vi "Create Table.vi"(8 "error in (no error)":errorcluster, 11 "User DB in":refnum<class "User DB.lvclass">) -> (0 "error out":errorcluster, 3 "User DB out":refnum<class "User DB.lvclass">)   [LabVIEW 2020, in "Summer of LabVIEW.lvlib" / "User DB.lvclass"]
uses:
  User DB.lvclass
  User DB.lvclass/User DB.ctl
  <vilib>/drjdpowell/SQLite Library/SQL Connection/Execute SQL (No results).vi
  SQLite/SQLite.lvclass
  <vilib>/drjdpowell/SQLite Library/SQLite.lvlib
  <vilib>/drjdpowell/SQLite Library/SQL Connection/Connection.lvclass
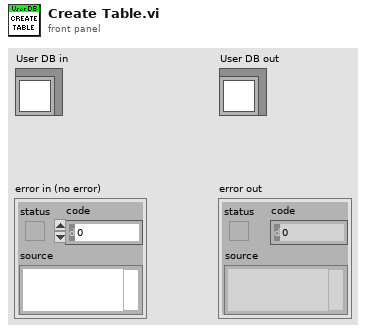
[diagram p1: front panel]
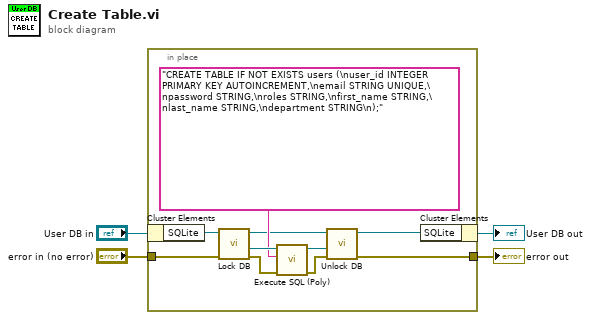
[diagram p0: block diagram]
diagram:
  n1 = in-place {
    in-place-border: "error in (no error)" -> [w13]
    in-place-border: [w5] -> w2
    n2 = in-place-cluster #1("User DB in") -> ("SQLite"=w14:refnum<class "SQLite.lvclass">)
    n3 = call "Lock DB.vi"("error in (no error)"=w13, "SQLite in"=w14) -> ("error out"=w11:errorcluster, "SQLite DB"=w12:refnum<class "Connection.lvclass">, "SQLite out"=w9:refnum<class "SQLite.lvclass">)  [unwired: 6 in, 1 out]
    n4 = call-poly <vilib>:"Execute SQL (Poly).vi"("error in (no error)"=w11, "SQL"="CREATE TABLE IF NOT EXISTS users (\nuser_id INTEGER PRIMARY KEY AUTOINCREMENT,\nemail STRING UNIQUE,\npassword STRING,\nroles STRING,\nfirst_name STRING,\nlast_name STRING,\ndepartment STRING\n);", "SQLite Connection in"=w12) -> ("error out"=w8:errorcluster, "SQLite Connection"=w7:refnum<class "Connection.lvclass">)  [unwired: 7 in]
    n5 = call "Unlock DB.vi"("error in (no error)"=w8, "SQLite DB"=w7, "SQLite in"=w9) -> ("error out"=w5:errorcluster, "SQLite out"=w6:refnum<class "SQLite.lvclass">)  [unwired: 7 in]
    n6 = in-place-cluster #1("SQLite"=w6) -> (→"User DB out":refnum<class "User DB.lvclass">)
  }
  "error out" <- w2
